vi "例程07-数字滤波器.vi"() -> ()   [LabVIEW 2016]
uses:
  <vilib>/measure/NI_MABase.lvlib
panel:
  out "Filtered Signal":dynamicdata(graph) caption="滤波后的信号"
  in  "phase":dbl caption="相位" format="%.2p"
  in  "amplitude":dbl=1.0 caption="幅值" format="%0.2p"
  in  "frequency":dbl=10.0 caption="频率" format="%0.2p"
  in  "停止":bool
  out "波形图":waveform(dbl)(graph)
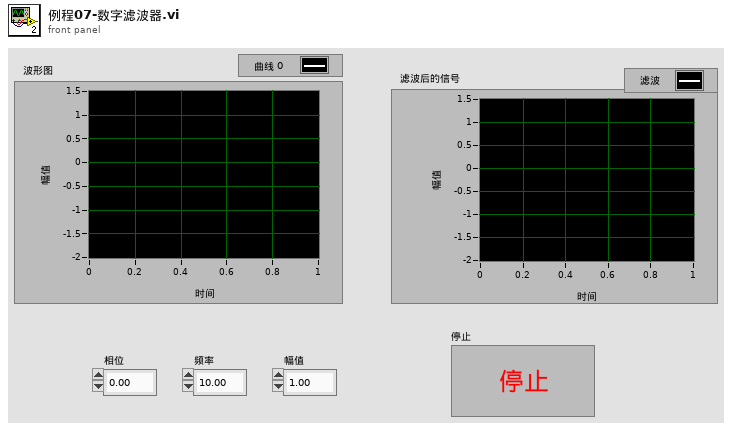
[diagram p1: front panel]
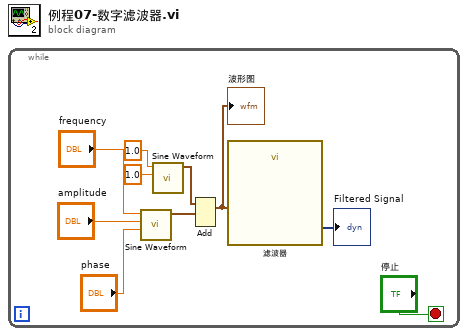
[diagram p0: block diagram]
diagram:
  n1 = while {
    stop <- "停止" stop-if-true
    n2 = call <vilib>:"Sine Waveform.vi"("phase"="phase", "amplitude"="amplitude", "frequency"="frequency") -> ("signal out"=w3:waveform(dbl))  [unwired: 7 in, 1 out]
    n3 = call <vilib>:"Sine Waveform.vi"("amplitude"=1.0, "frequency"=1.0) -> ("signal out"=w4:waveform(dbl))  [unwired: 8 in, 1 out]
    n4 = Add(1:w3, 2:w4) -> (0:w2:waveform(dbl))  [unwired: 1 in, 1 out]
    "波形图" <- w2
    n5 = call "滤波器"("Signal"=w2) -> ("Filtered Signal"=→"Filtered Signal":dynamicdata)  [unwired: 9 in, 1 out]
  }
